vi "loadFile.vi"(11 "String 2":string="QAMT01\\CRH3605") -> (0 "String":string, 2 "f":bool)   [LabVIEW 2012]
panel:
  out "concatenated string 3":string
  out "concatenated string 2":string
  out "standard output 5":string
  out "standard output 4":string
  out "text":string
  out "after substring":string
  out "before substring":string
  out "concatenated string":string
  out "standard output 3":string
  out "standard error 2":string
  out "error out":errorcluster
  in  "error in (no error)":errorcluster
  out "standard output 2":string
  out "standard error":string
  out "standard output":string
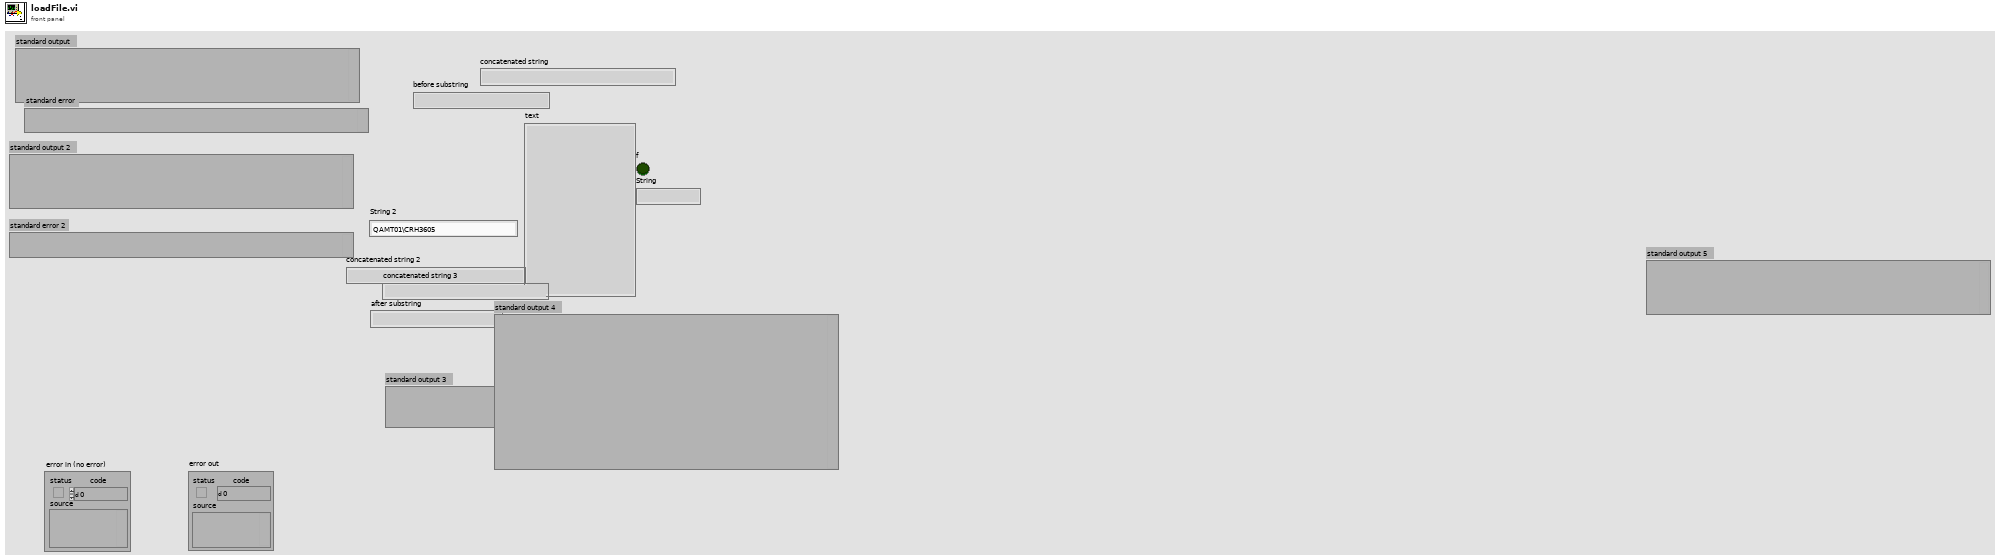
[diagram p1: front panel]
types:
  T1 = enum16{"open", "replace", "create", "open or create", "replace or create", "replace or create with confirmation"}
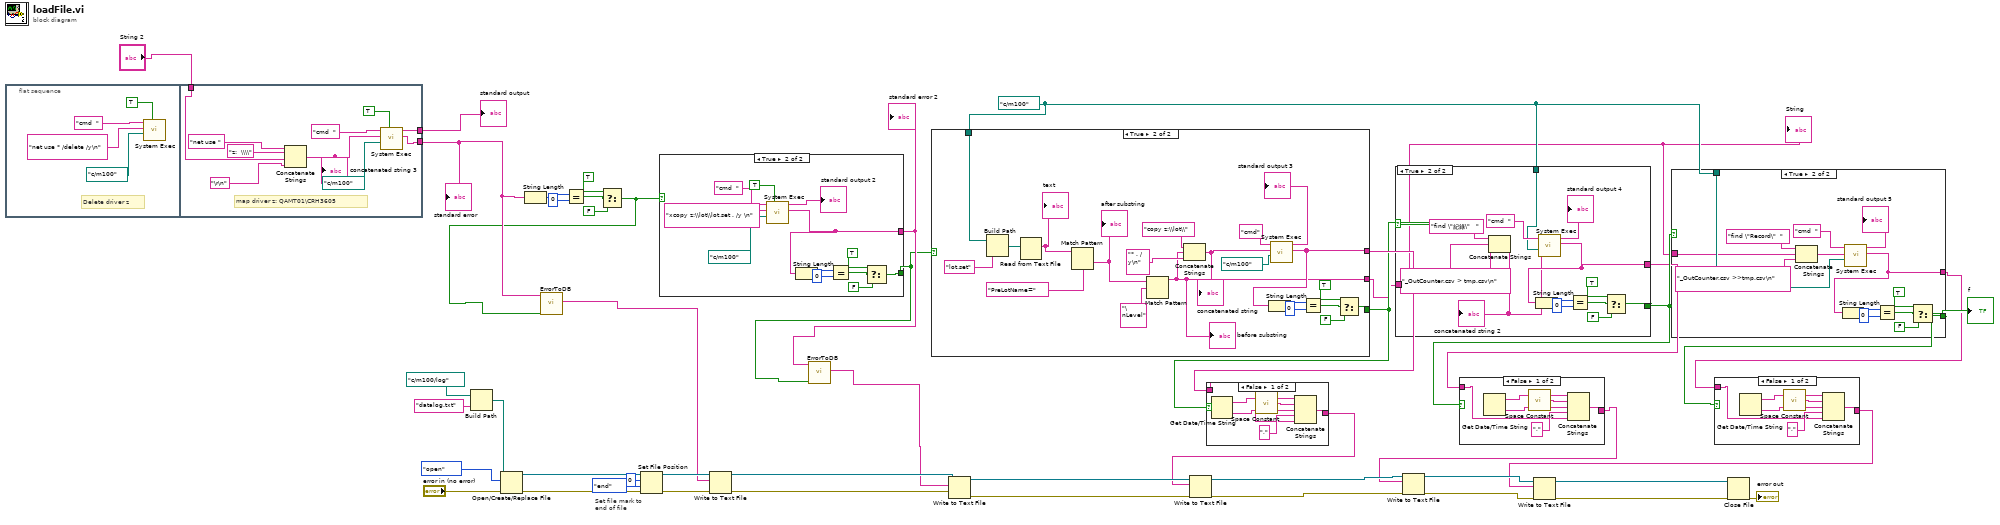
[diagram p0: block diagram]
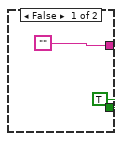
[diagram p4: hidden frame]
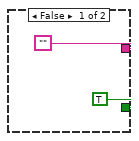
[diagram p5: hidden frame]
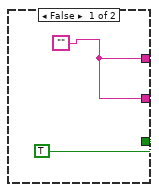
[diagram p7: hidden frame]
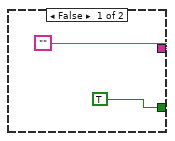
[diagram p8: hidden frame]
diagram:
  w21 = path "c:/m100" ("base path")
  # "Set file mark to\nend of file"
  n1 = flat-sequence {
    tunnel: [w55] -> w27
    tunnel: [w54] -> w5
    tunnel: "String 2" -> [w52]
    frame #0 {
      # "Delete driver z"
      n2 = call <vilib>:"System Exec.vi"("wait until completion? (T)"=TRUE, "working directory"=path "c:/m100", "standard input"="net use * /delete /y\n" ("string"), "command line"="cmd  ") -> ()  [unwired: 2 in, 6 out]
    }
    frame #1 {
      # "map driver z: QAMT01\\CRH3605"
      n3 = Concatenate Strings("net use " ("string"), "z:  \\\\" ("string"), w52, "\r\n") -> (w60:string)
      "concatenated string 3" <- w60
      n4 = call <vilib>:"System Exec.vi"("wait until completion? (T)"=TRUE, "working directory"=path "c:/m100", "standard input"=w60, "command line"="cmd  ") -> ("standard error"=w54:string, "standard output"=w55:string)  [unwired: 2 in, 4 out]
    }
  }
  n5 = Build Path(base path=path "c:/m100/log" ("path"), name or relative path="datalog.txt") -> (appended path=w30:path)
  n6 = Open/Create/Replace File(file path (use dialog)=w30, error in="error in (no error)", operation (0:open)=T1."open") -> (refnum out=w35:refnum<file>, error out=w34:errorcluster)  [unwired: 3 in, 1 out]
  n7 = String Length(string=w5) -> (length=w46:i32)
  n8 = Equal?(x=w46, y=0) -> (x = y?=w44:bool)
  n9 = Select(t=TRUE, s=w44, f=FALSE) -> (s? t:f=w4:bool)
  n10 = call "ErrorToDB.vi"("Error"=w4, "Error Message"=w5) -> ("LogData"=w6:string)  [unwired: 9 in]
  n11 = Set File Position(offset (in bytes) (0)=i64 0, refnum=w35, from (0:start)=enum16{"start", "end", "current"}."end", error in=w34) -> (refnum out=w37:refnum<file>, error out=w38:errorcluster)
  n12 = case shown="True" w4 {
    tunnel: [TRUE w64] -> w1
    tunnel: ["" w63] -> w2
    frame False {
    }
    frame True {
      n13 = call <vilib>:"System Exec.vi"("wait until completion? (T)"=TRUE, "working directory"=path "c:/m100", "standard input"="xcopy z:\\lot\\lot.set . /y \n", "command line"="cmd  ") -> ("standard error"=w63:string, "standard output"=→"standard output 2":string)  [unwired: 2 in, 4 out]
      n14 = String Length(string=w63) -> (length=w70:i32)
      n15 = Equal?(x=w70, y=0) -> (x = y?=w72:bool)
      n16 = Select(t=TRUE, s=w72, f=FALSE) -> (s? t:f=w64:bool)
    }
  }
  "standard error 2" <- w2
  n17 = Write to Text File(file (use dialog)=w37, text=w6, error in=w38) -> (refnum out=w29:refnum<file>, error out=w28:errorcluster)  [unwired: 1 in, 1 out]
  n18 = call "ErrorToDB.vi"("Error"=w1, "Error Message"=w2) -> ("LogData"=w3:string)  [unwired: 9 in]
  n19 = case shown="True" w1 {
    tunnel: [TRUE w81] -> w22
    tunnel: [w75 w80] -> w23
    tunnel: w21 -> [_ w78]
    tunnel: [w75 w77] -> w9
    frame False {
      w75 = ""
    }
    frame True {
      n20 = Build Path(base path=w78, name or relative path="lot.set") -> (appended path=w97:path)
      n21 = Read from Text File(file (use dialog)=w97) -> (text=w94:string)  [unwired: 3 in, 3 out]
      "text" <- w94
      n22 = Match Pattern(string=w94, regular expression="PreLotName=") -> (after substring=w88:string)  [unwired: 1 in, 3 out]
      "after substring" <- w88
      n23 = Match Pattern(string=w88, regular expression="\nLevel") -> (before substring=w77:string)  [unwired: 1 in, 3 out]
      "before substring" <- w77
      n24 = Concatenate Strings("copy z:\\lot\\" ("string"), w77, "* . /y\n" ("string")) -> (w87:string)
      "concatenated string" <- w87
      n25 = call <vilib>:"System Exec.vi"("working directory"=path "c:/m100", "standard input"=w87, "command line"="cmd") -> ("standard error"=w80:string, "standard output"=→"standard output 3":string)  [unwired: 3 in, 4 out]
      n26 = String Length(string=w80) -> (length=w82:i32)
      n27 = Equal?(x=w82, y=0) -> (x = y?=w84:bool)
      n28 = Select(t=TRUE, s=w84, f=FALSE) -> (s? t:f=w81:bool)
    }
  }
  "String" <- w9
  n29 = Write to Text File(file (use dialog)=w29, text=w3, error in=w28) -> (refnum out=w25:refnum<file>, error out=w26:errorcluster)  [unwired: 1 in, 1 out]
  n30 = case shown="False" w22 {
    tunnel: [w99 w104] -> w24
    tunnel: w23 -> [w98 w104]
    frame False {
      n31 = Get Date/Time String() -> (date string=w101:string, time string=w102:string)  [unwired: 3 in]
      n32 = call <vilib>:"Space Constant.vi"() -> ("String"=w100:string)
      n33 = Concatenate Strings(w101, w100, w102, "," ("string"), w98) -> (w99:string)
    }
    frame True {
    }
  }
  n34 = Write to Text File(file (use dialog)=w25, text=w24, error in=w26) -> (refnum out=w17:refnum<file>, error out=w16:errorcluster)  [unwired: 1 in, 1 out]
  n35 = case shown="True" w22 {
    tunnel: [TRUE w113] -> w20
    tunnel: ["" w112] -> w19
    tunnel: w9 -> [_ w110]
    tunnel: w21 -> [_ w107]
    frame False {
    }
    frame True {
      n36 = Concatenate Strings("find \"紀錄\"   " ("string"), w110, "_OutCounter.csv > tmp.csv\n" ("string")) -> (w108:string)
      "concatenated string 2" <- w108
      n37 = call <vilib>:"System Exec.vi"("working directory"=w107, "standard input"=w108, "command line"="cmd  ") -> ("standard error"=w112:string, "standard output"=→"standard output 4":string)  [unwired: 3 in, 4 out]
      n38 = String Length(string=w112) -> (length=w116:i32)
      n39 = Equal?(x=w116, y=0) -> (x = y?=w118:bool)
      n40 = Select(t=TRUE, s=w118, f=FALSE) -> (s? t:f=w113:bool)
    }
  }
  n41 = case shown="False" w20 {
    tunnel: [w122 w127] -> w15
    tunnel: w19 -> [w121 w127]
    frame False {
      n42 = Get Date/Time String() -> (date string=w124:string, time string=w125:string)  [unwired: 3 in]
      n43 = call <vilib>:"Space Constant.vi"() -> ("String"=w123:string)
      n44 = Concatenate Strings(w124, w123, w125, "," ("string"), w121) -> (w122:string)
    }
    frame True {
    }
  }
  n45 = Write to Text File(file (use dialog)=w17, text=w15, error in=w16) -> (refnum out=w14:refnum<file>, error out=w12:errorcluster)  [unwired: 1 in, 1 out]
  n46 = case shown="True" w20 {
    tunnel: [TRUE w136] -> w18
    tunnel: w21 -> [_ w132]
    tunnel: w9 -> [_ w131]
    tunnel: ["" w130] -> w7
    frame False {
    }
    frame True {
      n47 = Concatenate Strings("find \"Record\"  " ("string"), w131, "_OutCounter.csv >>tmp.csv\n" ("string")) -> (w133:string)
      n48 = call <vilib>:"System Exec.vi"("working directory"=w132, "standard input"=w133, "command line"="cmd  ") -> ("standard error"=w130:string, "standard output"=→"standard output 5":string)  [unwired: 3 in, 4 out]
      n49 = String Length(string=w130) -> (length=w139:i32)
      n50 = Equal?(x=w139, y=0) -> (x = y?=w141:bool)
      n51 = Select(t=TRUE, s=w141, f=FALSE) -> (s? t:f=w136:bool)
    }
  }
  "f" <- w18
  n52 = case shown="False" w18 {
    tunnel: [w145 w150] -> w10
    tunnel: w7 -> [w144 w150]
    frame False {
      n53 = Get Date/Time String() -> (date string=w147:string, time string=w148:string)  [unwired: 3 in]
      n54 = call <vilib>:"Space Constant.vi"() -> ("String"=w146:string)
      n55 = Concatenate Strings(w147, w146, w148, "," ("string"), w144) -> (w145:string)
    }
    frame True {
    }
  }
  n56 = Write to Text File(file (use dialog)=w14, text=w10, error in=w12) -> (refnum out=w13:refnum<file>, error out=w11:errorcluster)  [unwired: 1 in, 1 out]
  n57 = Close File(refnum=w13, error in=w11) -> (error out=→"error out":errorcluster)  [unwired: 1 out]
  "standard output" <- w27
  "standard error" <- w5
